vi "Hash string.vi"(3 "input string":string) -> (1 "Hash":i32)   [LabVIEW 2021, in "MatS Libs.lvlib"]
uses:
  <userlib>/MatS Libs/MatS Libs.lvlib
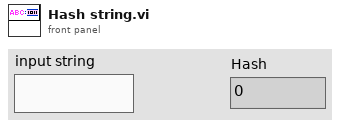
[diagram p1: front panel]
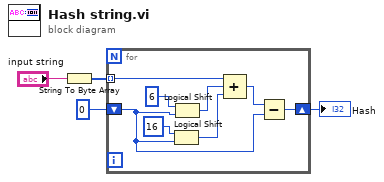
[diagram p0: block diagram]
diagram:
  n1 = String To Byte Array(string="input string") -> (unsigned byte array=w4:u8[])
  n2 = for {
    tunnel: w4 -> [w12] mode=indexing
    shift-right: [w5] -> w1
    shift-left: 0 -> [w6]
    n3 = Logical Shift(y=i16 16, x=w6) -> (x << y=w8:i32)
    n4 = Logical Shift(y=i16 6, x=w6) -> (x << y=w10:i32)
    n5 = Compound Arithmetic op=ADD(w12, w10, w8) -> (w7:i32)
    n6 = Subtract(x=w7, y=w6) -> (x-y=w5:i32)
  }
  "Hash" <- w1
